vi "Make Drink.vi"(8 "error in (no error)":errorcluster, 10 "Order Item in":refnum<class "Order Item.lvclass">, 11 "Barista in":refnum<class "Barista.lvclass">) -> (0 "error out":errorcluster, 1 "Description":string, 2 "Order Item out":refnum<class "Order Item.lvclass">, 3 "Barista out":refnum<class "Barista.lvclass">)   [LabVIEW 2023, in "Barista.lvclass"]
doc: "Simulates creation of a drink by the barista."
uses:
  Barista.lvclass
  Order/Order Item.lvclass
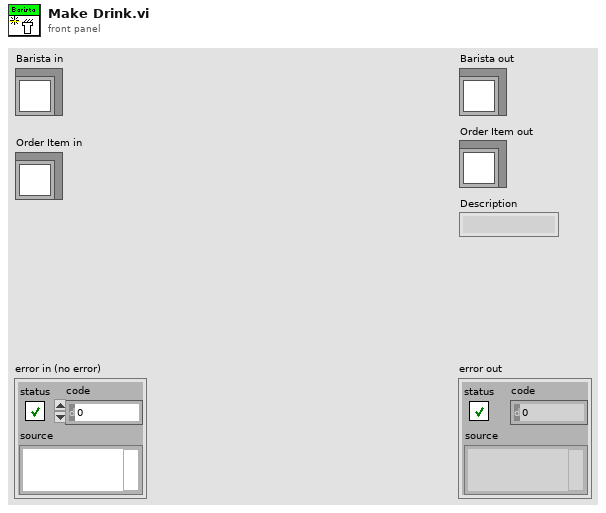
[diagram p1: front panel]
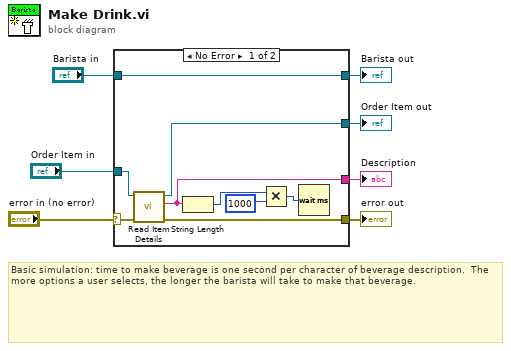
[diagram p0: block diagram]
diagram:
  # "Basic simulation: time to make beverage is one second per character of beverage description.  The more options a user selects, the longer the barista will take to make that beverage."
  n1 = case shown="No Error" "error in (no error)" {
    selector: "error in (no error)" -> [w15 w19]
    tunnel: [w10 w19] -> w6
    tunnel: [w16 w18] -> w4
    tunnel: "Barista in" -> [w16 w18]
    tunnel: "Order Item in" -> [w14 w17]
    tunnel: [w9 w17] -> w2
    tunnel: [w8 _] -> w1
    frame No Error {
      n2 = call-dynamic "Read Item Details.vi"("error in (no error)"=w15, "Order Item in"=w14) -> ("error out"=w10:errorcluster, "Description"=w8:string, "Order Item out"=w9:refnum<class "Order Item.lvclass">)  [unwired: 7 in]
      n3 = String Length(string=w8) -> (length=w13:i32)
      n4 = Multiply(x=w13, y=1000) -> (x*y=w11:i32)
      n5 = Wait (ms)(milliseconds to wait=w11) -> ()  [unwired: 1 out]
    }
    frame Error {
    }
  }
  "error out" <- w6
  "Barista out" <- w4
  "Order Item out" <- w2
  "Description" <- w1
